vi "Write Data.vi"(8 "error in (no error)":errorcluster, 10 "Data":u8[](array[numeric])=[0, 0, 0, 0, 0, 0, 0, 0, 0, 0, 0, 0, 0, 0, 0, 0, 0, 0, 0, 0, 0, 0, 0, 0, 0, 0, 0, 0, 0, 0, 0, 0], 11 "Serial Message in":refnum<class "Serial Message.lvclass">) -> (0 "error out":errorcluster, 3 "Serial Message out":refnum<class "Serial Message.lvclass">)   [LabVIEW 2013, in "Serial Message.lvclass"]
uses:
  Serial Message.lvclass
  Serial Message.lvclass/Serial Message.ctl
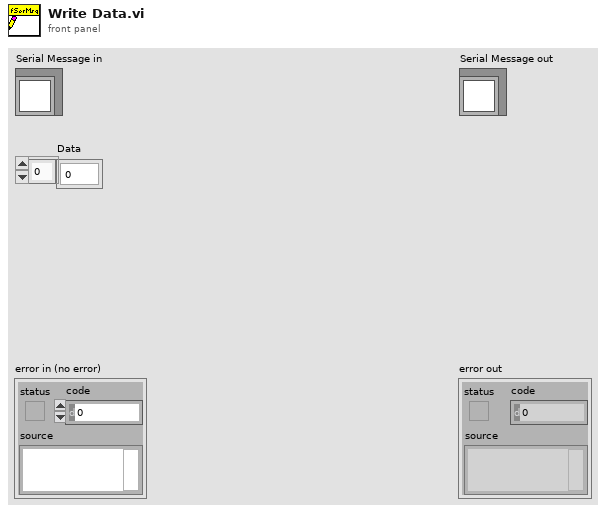
[diagram p1: front panel]
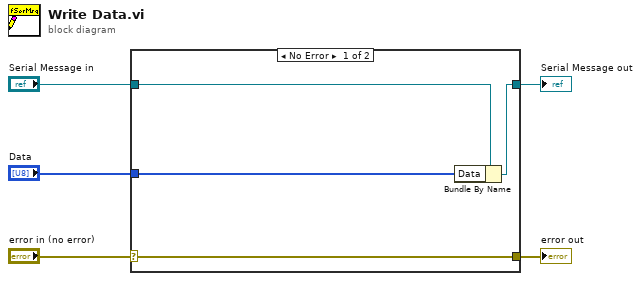
[diagram p0: block diagram]
diagram:
  n1 = case shown="No Error" "error in (no error)" {
    selector: "error in (no error)" -> [w9 w10]
    tunnel: [w9 w10] -> w4
    tunnel: [w7 w11] -> w2
    tunnel: "Serial Message in" -> [w8 w11]
    tunnel: "Data" -> [w6 _]
    frame No Error {
      n2 = Bundle By Name(cluster=w8, "Data"=w6) -> (w7:refnum<class "Serial Message.lvclass">)
    }
    frame Error {
    }
  }
  "error out" <- w4
  "Serial Message out" <- w2
